vi "Trace in Corners.vi"(10 "Start Vectors":T1, 11 "Map in":refnum<class "Maze.lvclass">) -> (3 "Map out":refnum<class "Maze.lvclass">)   [LabVIEW 2021, in "Maze.lvclass"]
uses:
  Maze.lvclass
  Position.ctl
  Maze.lvclass/Maze.ctl
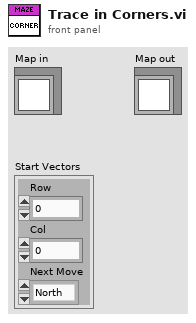
[diagram p1: front panel]
types:
  T1 = typedef "Maze.lvclass/Position.ctl" = cluster{"Row":u64, "Col":u64, "Next Move":enum16{"North", "East", "South", "West", "Halt"}}
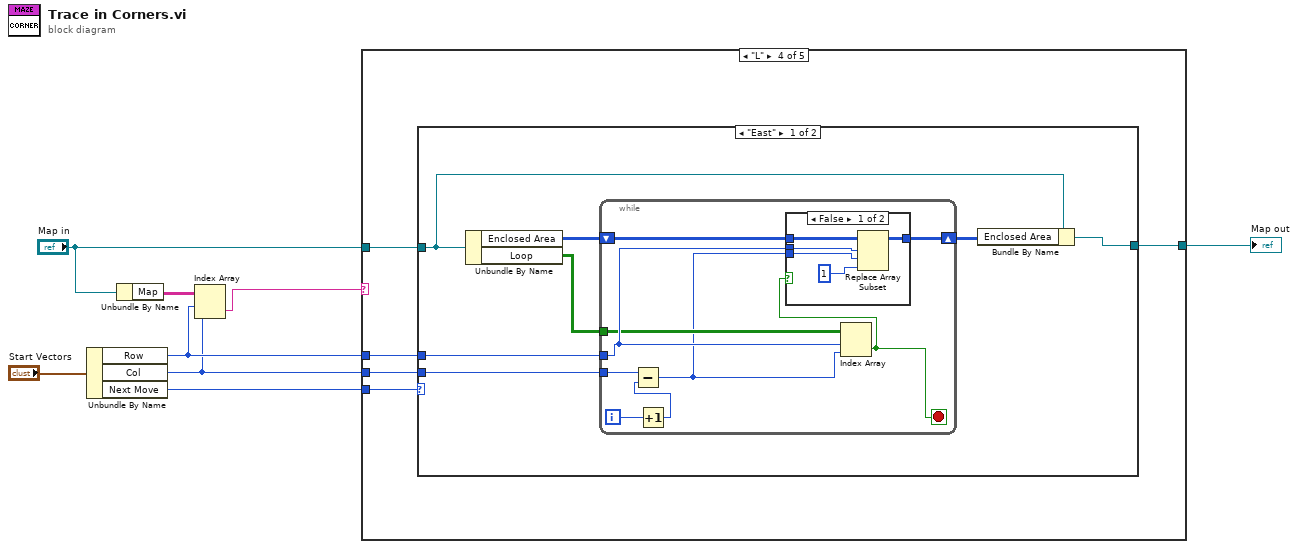
[diagram p0: block diagram]
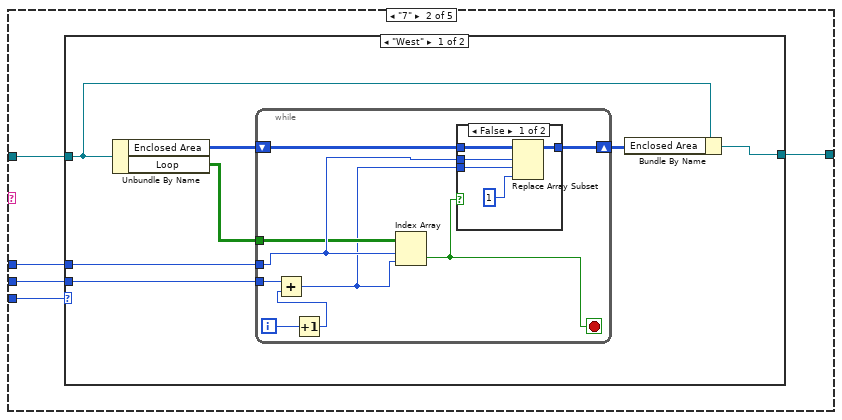
[diagram p3: hidden frame]
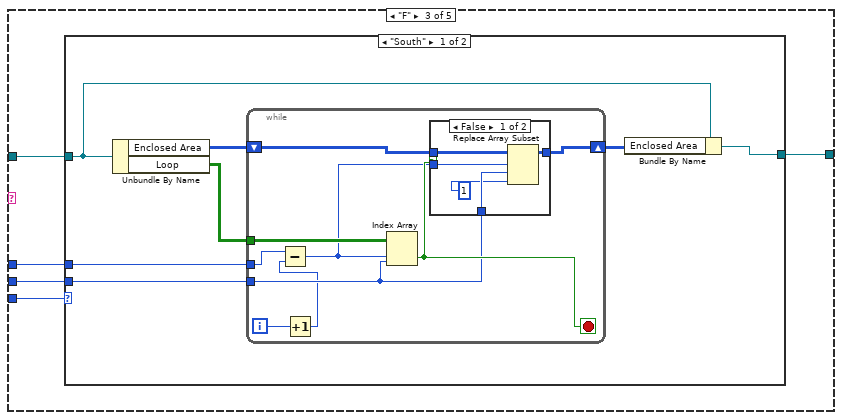
[diagram p6: hidden frame]
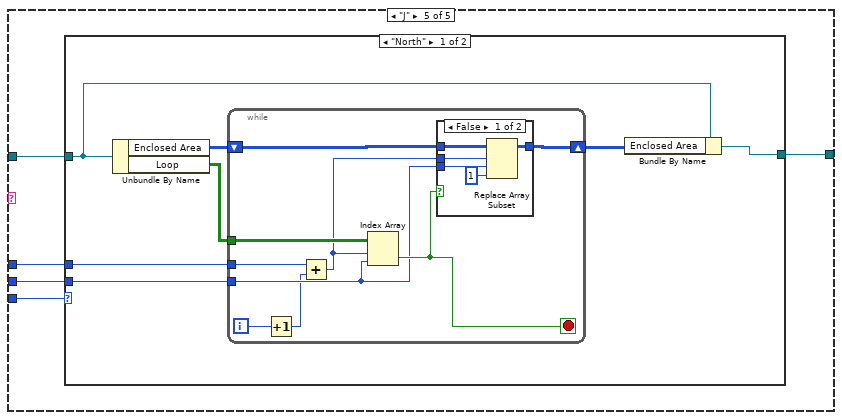
[diagram p11: hidden frame]
diagram:
  n1 = Unbundle By Name("Start Vectors") -> ("Row"=w2:u64, "Col"=w1:u64, "Next Move"=w3:enum16{"North", "East", "South", "West", "Halt"})
  n2 = Unbundle By Name("Map in") -> ("Map"=w7:string[][])
  n3 = Index Array(array=w7, index (row)=w2, index (col)=w1) -> (element=w6:string)
  n4 = case shown="\"L\"" w6 {
    tunnel: w3 -> [_ w14 w42 w70 w98]
    tunnel: [w9 w13 w41 w69 w97] -> w8
    tunnel: "Map in" -> [w9 w12 w40 w68 w96]
    tunnel: w2 -> [_ w11 w39 w67 w95]
    tunnel: w1 -> [_ w10 w38 w66 w94]
    frame Default {
    }
    frame "7" {
      n5 = case shown="\"West\"" w14 {
        tunnel: [w21 w37] -> w13
        tunnel: w12 -> [w20 w37]
        tunnel: w11 -> [w19 _]
        tunnel: w10 -> [w17 _]
        frame "West" {
          n6 = Unbundle By Name(w20) -> ("Enclosed Area"=w16:i32[][], "Loop"=w18:bool[][])
          n7 = while {
            tunnel: w19 -> [w30]
            tunnel: w18 -> [w28]
            tunnel: w17 -> [w24]
            shift-right: [w26] -> w15
            shift-left: w16 -> [w27]
            i -> [w29]
            stop <- w25 stop-if-true
            n8 = Increment(x=w29) -> (x+1=w22:i32)
            n9 = Add(x=w24, y=w22) -> (x+y=w23:u64)
            n10 = Index Array(array=w28, index (row)=w30, index (col)=w23) -> (element=w25:bool)
            n11 = case shown="False" w25 {
              tunnel: w30 -> [w35 _]
              tunnel: w27 -> [w34 w36]
              tunnel: [w33 w36] -> w26
              tunnel: w23 -> [w31 _]
              frame False {
                n12 = Replace Array Subset(array=w34, new element=1 ("new element/subarray"), index (row)=w35, index (col)=w31) -> (w33:i32[][])
              }
              frame True {
              }
            }
          }
          n13 = Bundle By Name(cluster=w20, "Enclosed Area"=w15) -> (w21:refnum<class "Maze.lvclass">)
        }
        frame Default {
        }
      }
    }
    frame "F" {
      n14 = case shown="\"South\"" w42 {
        tunnel: [w49 w65] -> w41
        tunnel: w40 -> [w48 w65]
        tunnel: w39 -> [w47 _]
        tunnel: w38 -> [w45 _]
        frame "South" {
          n15 = Unbundle By Name(w48) -> ("Enclosed Area"=w44:i32[][], "Loop"=w46:bool[][])
          n16 = while {
            tunnel: w47 -> [w52]
            tunnel: w46 -> [w57]
            tunnel: w45 -> [w53]
            shift-right: [w55] -> w43
            shift-left: w44 -> [w56]
            i -> [w58]
            stop <- w54 stop-if-true
            n17 = Increment(x=w58) -> (x+1=w50:i32)
            n18 = Subtract(x=w52, y=w50) -> (x-y=w51:u64)
            n19 = Index Array(array=w57, index (row)=w51, index (col)=w53) -> (element=w54:bool)
            n20 = case shown="False" w54 {
              tunnel: w56 -> [w63 w64]
              tunnel: w53 -> [w62 _]
              tunnel: [w61 w64] -> w55
              tunnel: w51 -> [w59 _]
              frame False {
                n21 = Replace Array Subset(array=w63, new element=1 ("new element/subarray"), index (row)=w59, index (col)=w62) -> (w61:i32[][])
              }
              frame True {
              }
            }
          }
          n22 = Bundle By Name(cluster=w48, "Enclosed Area"=w43) -> (w49:refnum<class "Maze.lvclass">)
        }
        frame Default {
        }
      }
    }
    frame "L" {
      n23 = case shown="\"East\"" w70 {
        tunnel: [w77 w93] -> w69
        tunnel: w68 -> [w76 w93]
        tunnel: w67 -> [w75 _]
        tunnel: w66 -> [w73 _]
        frame "East" {
          n24 = Unbundle By Name(w76) -> ("Enclosed Area"=w72:i32[][], "Loop"=w74:bool[][])
          n25 = while {
            tunnel: w75 -> [w86]
            tunnel: w74 -> [w84]
            tunnel: w73 -> [w82]
            shift-right: [w81] -> w71
            shift-left: w72 -> [w83]
            i -> [w85]
            stop <- w80 stop-if-true
            n26 = Increment(x=w85) -> (x+1=w78:i32)
            n27 = Subtract(x=w82, y=w78) -> (x-y=w79:u64)
            n28 = Index Array(array=w84, index (row)=w86, index (col)=w79) -> (element=w80:bool)
            n29 = case shown="False" w80 {
              tunnel: w86 -> [w91 _]
              tunnel: w83 -> [w90 w92]
              tunnel: [w89 w92] -> w81
              tunnel: w79 -> [w87 _]
              frame False {
                n30 = Replace Array Subset(array=w90, new element=1 ("new element/subarray"), index (row)=w91, index (col)=w87) -> (w89:i32[][])
              }
              frame True {
              }
            }
          }
          n31 = Bundle By Name(cluster=w76, "Enclosed Area"=w71) -> (w77:refnum<class "Maze.lvclass">)
        }
        frame Default {
        }
      }
    }
    frame "J" {
      n32 = case shown="\"North\"" w98 {
        tunnel: [w105 w121] -> w97
        tunnel: w96 -> [w104 w121]
        tunnel: w95 -> [w103 _]
        tunnel: w94 -> [w101 _]
        frame "North" {
          n33 = Unbundle By Name(w104) -> ("Enclosed Area"=w100:i32[][], "Loop"=w102:bool[][])
          n34 = while {
            tunnel: w103 -> [w114]
            tunnel: w102 -> [w112]
            tunnel: w101 -> [w108]
            shift-right: [w110] -> w99
            shift-left: w100 -> [w111]
            i -> [w113]
            stop <- w109 stop-if-true
            n35 = Increment(x=w113) -> (x+1=w106:i32)
            n36 = Add(x=w114, y=w106) -> (x+y=w107:u64)
            n37 = Index Array(array=w112, index (row)=w107, index (col)=w108) -> (element=w109:bool)
            n38 = case shown="False" w109 {
              tunnel: w111 -> [w119 w120]
              tunnel: w107 -> [w118 _]
              tunnel: w108 -> [w117 _]
              tunnel: [w116 w120] -> w110
              frame False {
                n39 = Replace Array Subset(array=w119, new element=1 ("new element/subarray"), index (row)=w118, index (col)=w117) -> (w116:i32[][])
              }
              frame True {
              }
            }
          }
          n40 = Bundle By Name(cluster=w104, "Enclosed Area"=w99) -> (w105:refnum<class "Maze.lvclass">)
        }
        frame Default {
        }
      }
    }
  }
  "Map out" <- w8
